vi "Press_Test.vi"() -> (2 "Reset Button":bool)   [LabVIEW 2014]
uses:
  <vilib>/Platform/TimedLoop/XDataNode/timing_clust.ctl
  <vilib>/Platform/TimedLoop/XDataNode/nitl_modes.ctl
  <vilib>/Platform/TimedLoop/XDataNode/wakeup.ctl
  <vilib>/Platform/TimedLoop/XDataNode/XDataNode.xnode
  <vilib>/Platform/TimedLoop/XDataNode/XDNodeRunTimeDep.lvlib
panel:
  out "Time":dbl
  out "Pass":bool
  out "Fail":bool
  in  "OK Button":bool
  out "Pressure":dynamicdata(graph)
  # "s"
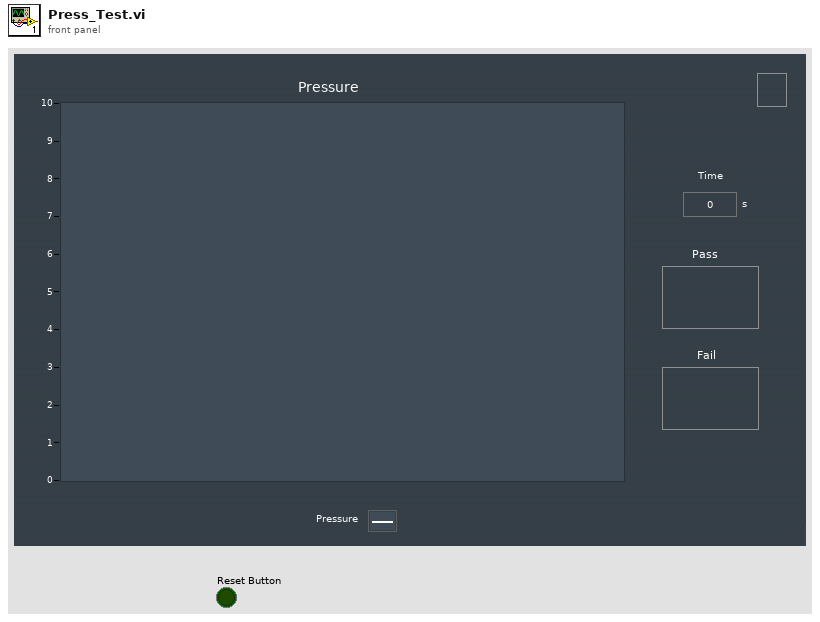
[diagram p1: front panel]
types:
  T1 = typedef "XDNodeRunTimeDep.lvlib/timing_clust.ctl" = cluster{"Expected End [f-1]":u64, "Actual End [f-1]":u64, "Finished Late? [f-1]":bool, "Expected End [i-1]":u64, "Actual End [i-1]":u64, "Finished Late? [i-1]":bool, "Expected Start [i]":u64, "Actual Start [i]":u64, "Expected Start [f]":u64, "Actual Start [f]":u64, "Source Name":string, "Structure Name":string, "Period":i64, "Deadline":i64, "Offset":i64, "Start":i64, "Priority":i32, "Timeout":i32, "Mode":T2, "Wakeup Reason":T3, "Error":errorcluster, "Source Type":string, "Secondary Source Type":string, "Global End Time":u64, "Global Start Time":u64, "Frame Duration":u64, "Iteration Duration":u64, "Assigned CPU":i32, "I/O Scan Engine Mode":u32}
  T2 = typedef "XDNodeRunTimeDep.lvlib/nitl_modes.ctl" = enum32{"No Change", "Process missed periods, maintain original phase", "Discard missed periods, maintain original phase", "Process missed periods, ignore original phase", "Discard missed periods, ignore original phase"}
  T3 = typedef "XDNodeRunTimeDep.lvlib/wakeup.ctl" = enum32{"Normal", "Aborted", "Asynchronous wakeup", "Timing source error", "Timed loop error", "Timeout"}
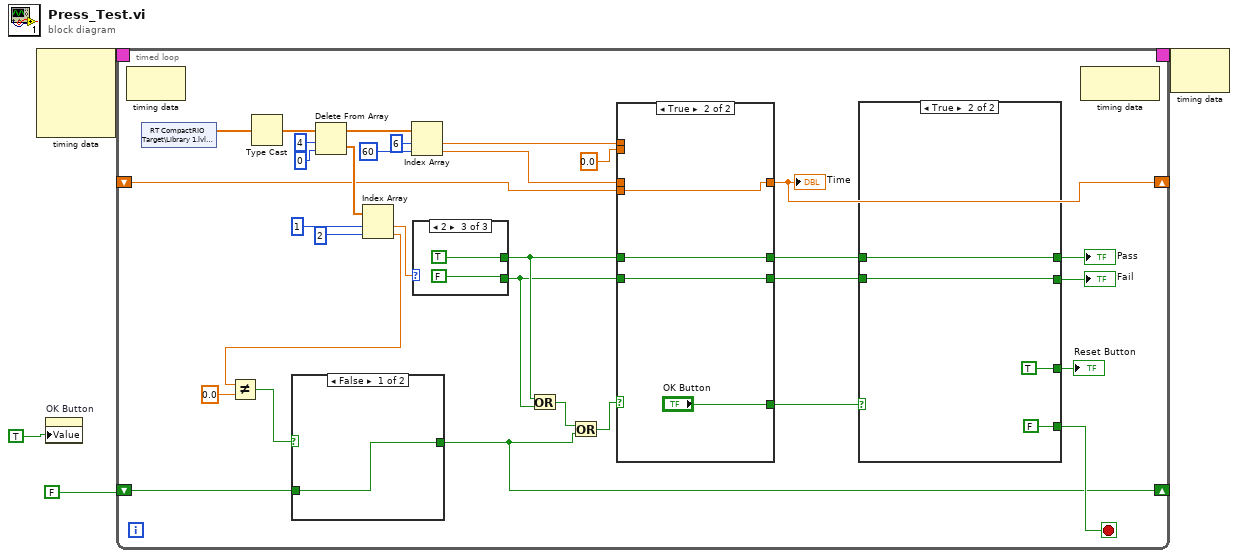
[diagram p0: block diagram]
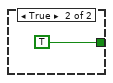
[diagram p2: hidden frame]
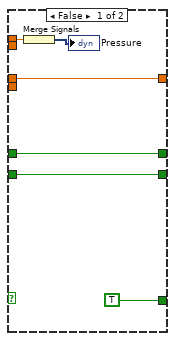
[diagram p3: hidden frame]
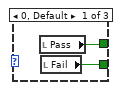
[diagram p4: hidden frame]
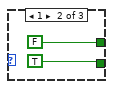
[diagram p5: hidden frame]
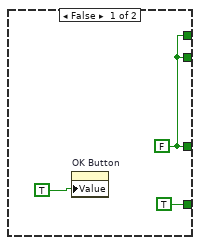
[diagram p6: hidden frame]
diagram:
  n1 = node-c288() -> (w4:T1)  [unwired: 4 in]
  n2 = property on="OK Button" class="Bool (strict)"("Value"=TRUE) -> ()  [unwired: 2 in, 2 out]
  n3 = timed-loop {
    timing: w4 -> [_]
    timing-out: [_] -> w3
    shift-right: [w14] -> _
    shift-left: _ -> [w13]
    shift-right: [w11] -> _
    shift-left: FALSE -> [w10]
    stop <- w36 stop-if-true
    n4 = node-c288() -> ()  [unwired: 1 in, 1 out]
    n5 = shared-variable "RT CompactRIO Target\\Library 1.lvlib\\DATA"() -> (w31:dbl[])  [unwired: 1 in, 1 out]
    n6 = Type Cast(type=w31, x=w31) -> (*(type *) &x=w32:dbl[])
    n7 = Delete From Array(array=w32, length=4, index=0) -> (deleted portion=w27:dbl[], array with subset deleted=w29:dbl[])
    n8 = Index Array(array=w27, index #1=1 ("index"), index #2=2 ("index")) -> (element #1=w25:dbl, element #2=w7:dbl)
    n9 = Not Equal?(x=w7, y=0.0) -> (x != y?=w6:bool)
    n10 = case shown="False" w6 {
      tunnel: [w37 TRUE] -> w11
      tunnel: w10 -> [w37 _]
      frame False {
      }
      frame True {
      }
    }
    n11 = Index Array(array=w29, index #1=6 ("index"), index #2=60 ("index")) -> (element #1=w24:dbl, element #2=w15:dbl)
    n12 = case shown="2" w25 {
      tunnel: [w49 TRUE FALSE] -> w18
      tunnel: [w50 FALSE TRUE] -> w20
      frame 0, Default {
        n13 = local read "Pass"() -> (w50:bool)
        n14 = local read "Fail"() -> (w49:bool)
      }
      frame 1 {
      }
      frame 2 {
      }
    }
    n15 = Or(x=w20, y=w18) -> (x .or. y?=w12:bool)
    n16 = Or(x=w12, y=w11) -> (x .or. y?=w5:bool)
    n17 = case shown="True" w5 {
      tunnel: [TRUE ("OK Button") "OK Button"] -> w35
      tunnel: w24 -> [w42 _]
      tunnel: 0.0 -> [_ _]
      tunnel: [w41 w47] -> w19
      tunnel: w20 -> [w41 w47]
      tunnel: w18 -> [w40 w46]
      tunnel: [w40 w46] -> w17
      tunnel: w15 -> [w39 _]
      tunnel: [w39 w45] -> w14
      tunnel: w13 -> [_ w45]
      frame False {
        n18 = Merge Signals(w42) -> (→"Pressure":dynamicdata)
      }
      frame True {
      }
    }
    "Time" <- w14
    n19 = case shown="True" w35 {
      tunnel: [TRUE FALSE] -> w36
      tunnel: [w55 TRUE] -> w28
      tunnel: [w55 w59] -> w22
      tunnel: [w55 w58] -> w21
      tunnel: w19 -> [_ w59]
      tunnel: w17 -> [_ w58]
      frame False {
        w55 = FALSE
        n20 = property on="OK Button" class="Bool (strict)"("Value"=TRUE) -> ()  [unwired: 2 in, 2 out]
      }
      frame True {
      }
    }
    "Reset Button" <- w28
    "Pass" <- w22
    "Fail" <- w21
    n21 = node-c288() -> ()  [unwired: 1 in, 1 out]
  }
  n22 = node-c288(w3) -> ()  [unwired: 1 out]
